vi "set_synth_state.vi"() -> ()   [LabVIEW 2014]
panel:
  in  "DC Val":dbl=175.0
  in  "Frequency (Hz)":dbl=175.0
  in  "DC?":bool=TRUE
  in  "Offset Trim (part per thousand)":i32
  in  "Auto Offset":bool=TRUE
  in  "Manual Offset (V)":dbl=175.0
  in  "Amplitude (V)":dbl=175.0
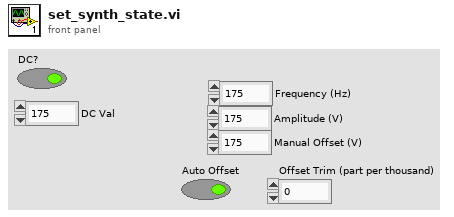
[diagram p1: front panel]
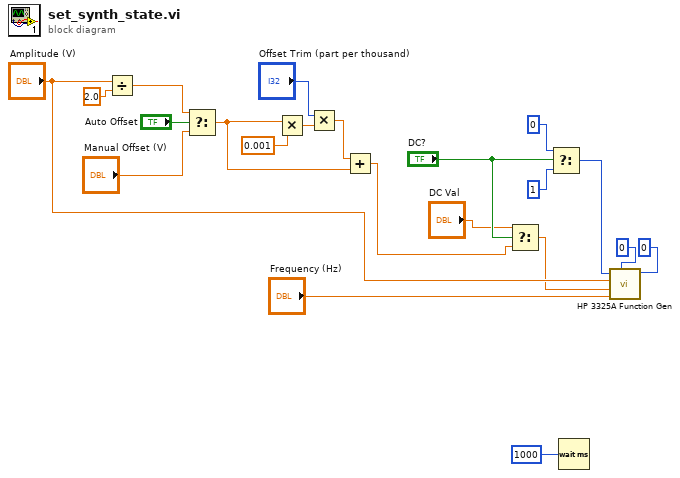
[diagram p0: block diagram]
diagram:
  n1 = Divide(x="Amplitude (V)", y=2.0) -> (x/y=w19:dbl)
  n2 = Select(t=w19, s="Auto Offset", f="Manual Offset (V)") -> (s? t:f=w17:dbl)
  n3 = Multiply(x=w17, y=0.001) -> (x*y=w14:dbl)
  n4 = Multiply(x="Offset Trim (part per thousand)", y=w14) -> (x*y=w13:dbl)
  n5 = Add(x=w13, y=w17) -> (x+y=w2:dbl)
  n6 = Select(t="DC Val", s="DC?", f=w2) -> (s? t:f=w1:dbl)
  n7 = Select(t=0, s="DC?", f=1) -> (s? t:f=w7:i32)
  n8 = Wait (ms)(milliseconds to wait=1000) -> ()  [unwired: 1 out]
  n9 = call "HP 3325A Function Gen.vi"("sweep function (none:0)"=0, "modulation (off:0)"=0, "frequency (Hz)"="Frequency (Hz)", "offset (V)"=w1, "amplitude (V)"="Amplitude (V)", "signal type (dc:0)"=w7) -> ()  [unwired: 4 in]
